vi "main.vi"(8 "Error in":errorcluster) -> (0 "error out":errorcluster)   [LabVIEW 2018, in "Sensor Interface.lvlib"]
doc: "The main VI of the module."
uses:
  Sensor Interface.lvlib
  vi/Module Queue Actions.ctl
  ctl/Module State--enum.ctl
  Common/Common.lvlib
  Common/ctl/Stop all modules states--enum.ctl
  Error Handler/Error Handler.lvlib
  Error Handler/ctl/Module State--enum.ctl
  Error Handler/ctl/Error source--enum.ctl
  Common/ctl/Error to pass.ctl
  Controller/Controller.lvlib
  Controller/ctl/Module State--enum.ctl
panel:
  in  "Funds Dispensed":bool
  in  "Deposit Received":bool
  # "Sensor Interface"
  # "[Covers: UI1]"
  # "[Covers: UI4]"
  # "[Covers: UI4A]"
  # "[Covers: UI4B]"
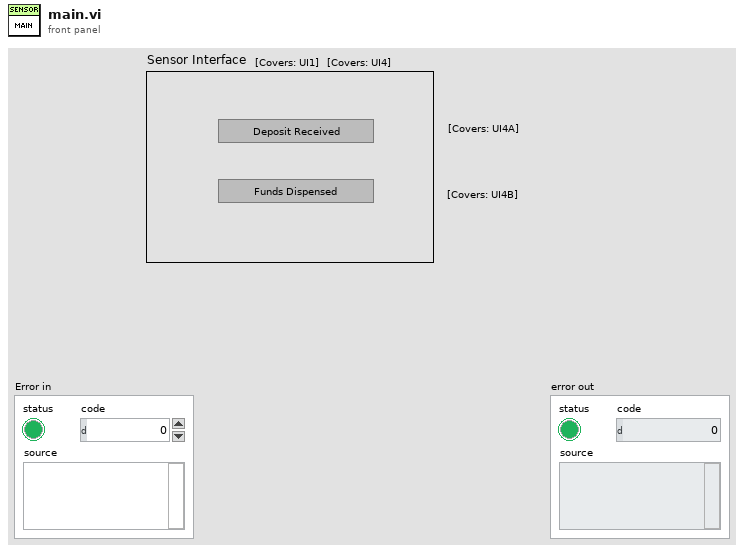
[diagram p1: front panel]
types:
  T1 = typedef "Sensor Interface.lvlib/Module Queue Actions.ctl" = enum16{"Create", "Get", "Destroy"}
  T2 = typedef "Common.lvlib/Stop all modules states--enum.ctl" = enum16{"Create", "Get", "Send 'Stop all' Message", "Destroy"}
  T3 = typedef "Sensor Interface.lvlib/Module State--enum.ctl" = enum16{"Init", "Error", "Idle", "Close", "Enable/disable controls"}
  T4 = typedef "Common.lvlib/Error source--enum.ctl" = enum16{"Display Console", "User Console", "Sensor Interface IO", "Process Step", "Other"}
  T5 = typedef "Common.lvlib/Error to pass.ctl" = cluster{"Error source":T4, "Error":errorcluster}
  T6 = typedef "Error Handler.lvlib/Module State--enum.ctl" = enum16{"Init", "Error", "Idle", "Close", "Handle External Error", "Log to file"}
  T7 = typedef "Controller.lvlib/Module State--enum.ctl" = enum16{"Init", "Error", "Close", "User Console: Card Reader Pressed", "Sensor Interface: Deposit Received pressed", "Sensor Interface: Funds Dispensed Pressed", "Idle", "Login State", "Balance Enquiry", "Deposit State", "Withdrawal State", "Fast Cash State", "Configuration Database", "Inactivity Timeout", "Terminate State", "Wait for account number", "Verify account number", "Wait for new transaction button"}
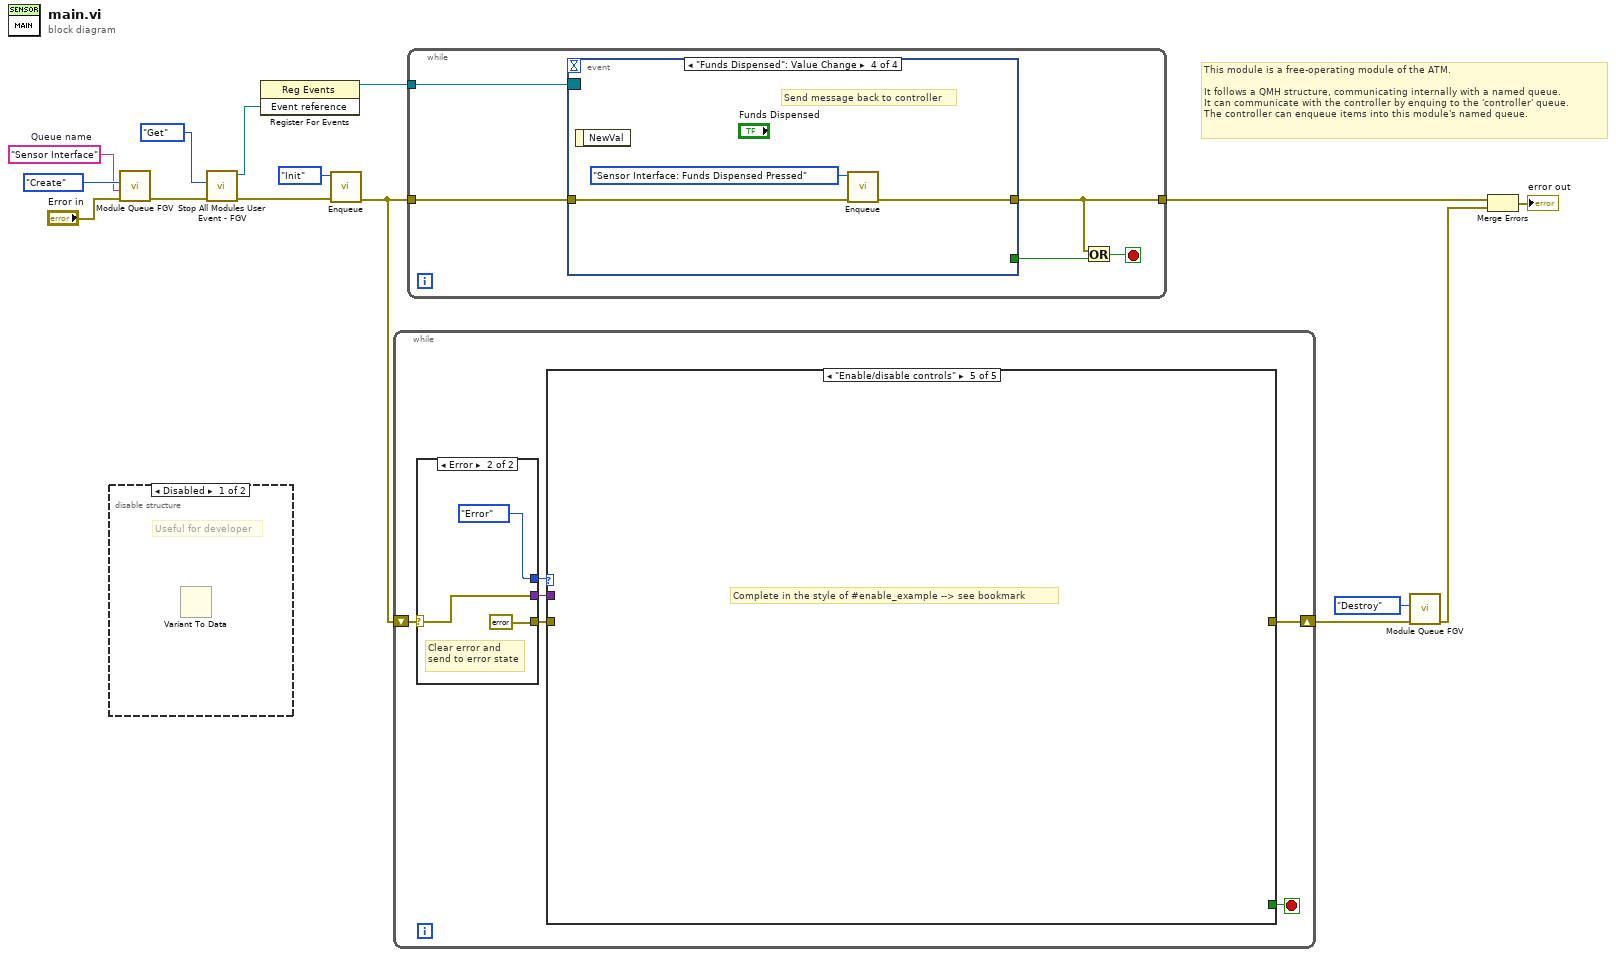
[diagram p0: block diagram]
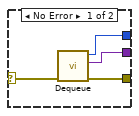
[diagram p3: hidden frame]
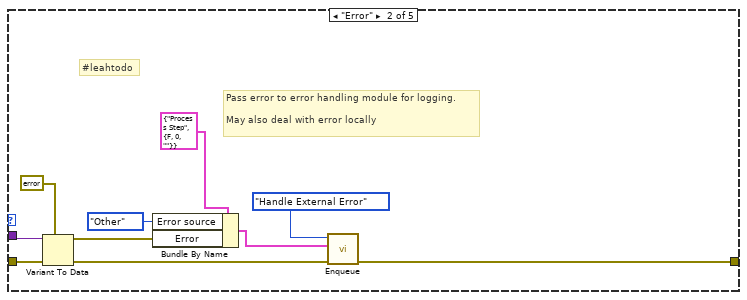
[diagram p5: hidden frame]
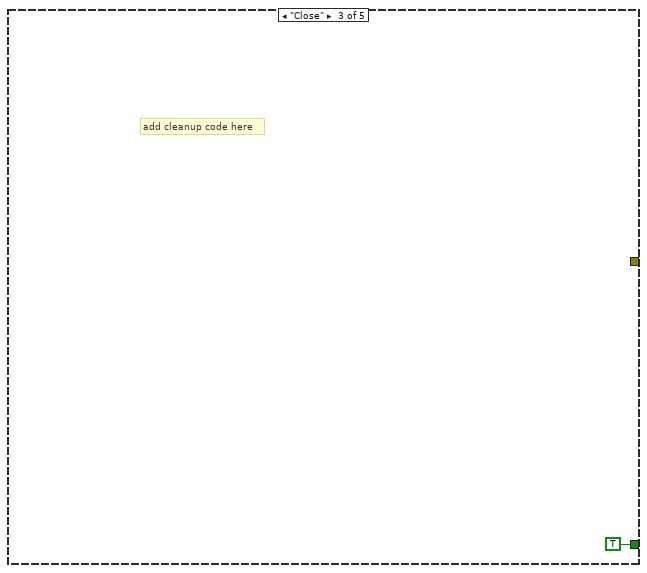
[diagram p6: hidden frame]
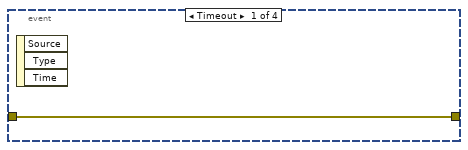
[diagram p8: hidden frame]
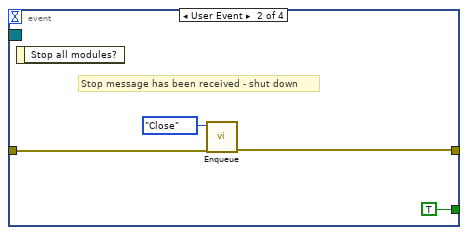
[diagram p9: hidden frame]
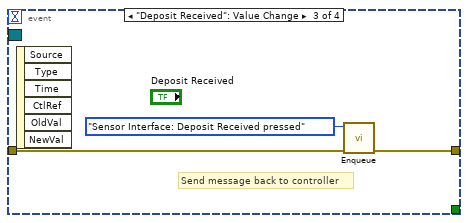
[diagram p10: hidden frame]
diagram:
  w14 = "Sensor Interface"  # Queue name
  # "This module is a free-operating module of the ATM.\n\nIt follows a QMH structure, communicating internally with a named queue.\nIt can communicate with the controller by enquing to the 'controller' queue.\nThe controller can enqueue items into this module's named queue."
  n1 = disable-structure shown="Disabled" {
    frame Disabled {
      # "Useful for developer"
      n2 = Variant To Data() -> ()  [unwired: 3 in, 2 out]
    }
    frame Enabled {
    }
  }
  n3 = call "Module Queue FGV.vi"("Error in"="Error in", "Queue name"=w14, "Module Queue Actions"=Module_Queue_Actions."Create") -> ("error out"=w9:errorcluster)  [unwired: 7 in, 1 out]
  n4 = call "Stop All Modules User Event - FGV.vi"("error in"=w9, "Action"=Stop_all_modules_states--enum."Get") -> ("error out"=w8:errorcluster, "Event reference"=w11:refnum<user-event>)  [unwired: 8 in]
  n5 = register-events(w11) -> (reference out=w10:refnum<event-registration>)  [unwired: 2 in, 1 out]
  n6 = call "Enqueue.vi"("error in (no error)"=w8, "State"=Module_State--enum."Init") -> ("error out"=w7:errorcluster)  [unwired: 9 in]
  n7 = while {
    shift-right: [w18] -> w5
    shift-left: w7 -> [w17]
    stop <- w16 stop-if-true
    n8 = case shown="Error" w17 {
      selector: w17 -> [w22 w27]
      tunnel: [w25 Module_State--enum."Error" ("State")] -> w21
      tunnel: [w24 w27] -> w20
      tunnel: [w23 errorcluster {"status"=FALSE, "code"=0, "source"=""} ("error out")] -> w19
      frame No Error {
        n9 = call "Dequeue.vi"("error in (no error)"=w22) -> ("error out"=w23:errorcluster, "Data"=w24:variant, "State"=w25:T3)  [unwired: 8 in]
      }
      frame Error {
        # "Clear error and\nsend to error state"
      }
    }
    n10 = case shown="\"Enable/disable controls\"" w21 {
      tunnel: w20 -> [_ w35 _ _ _]
      tunnel: w19 -> [_ w36 _ _ _]
      tunnel: [_ w37 _ _ _] -> w18
      tunnel: [_ _ TRUE _ _] -> w16
      frame "Init", Default {
        # "Disable both controls"
        # "[Covers: IS3]"
      }
      frame "Error" {
        # "#leahtodo"
        # "Pass error to error handling module for logging.\n\nMay also deal with error locally"
        n11 = Variant To Data(error in=w36, type=errorcluster {"status"=FALSE, "code"=0, "source"=""} ("error constant"), Variant=w35) -> (data=w31:errorcluster, error out=w33:errorcluster)
        n12 = Bundle By Name(cluster=T5 {"Error source"=enum."Process Step", "Error"={"status"=FALSE, "code"=0, "source"=""}} ("Error to pass"), "Error source"=Error_source--enum."Other", "Error"=w31) -> (w30:T5)
        n13 = call "Enqueue.vi"("error in (no error)"=w33, "Data"=w30, "State"=Module_State--enum."Handle External Error") -> ("error out"=w37:errorcluster)  [unwired: 8 in]
      }
      frame "Close" {
        # "add cleanup code here"
      }
      frame "Idle" {
      }
      frame "Enable/disable controls" {
        # "Complete in the style of #enable_example --> see bookmark"
      }
    }
  }
  n14 = while {
    tunnel: w7 -> [w44]
    tunnel: [w41] -> w3
    tunnel: w10 -> [w43]
    stop <- w42 stop-if-true
    n15 = event shown="[3] \"Funds Dispensed\": Value Change" {
      selector: w43 -> [_ _ _ _]
      dyn-events: _ -> [_ _ _ _]
      timeout: _ -> [_ _ _ _]
      tunnel: w44 -> [w45 w49 w51 w54]
      tunnel: [w45 w48 w50 w53] -> w41
      tunnel: [_ TRUE _ _] -> w40
      event Timeout {
        n16 = event-data() -> ()  [unwired: 1 in, 3 out]
      }
      event User Event {
        # "Stop message has been received - shut down"
        n17 = event-data() -> ()  [unwired: 1 in, 1 out]
        n18 = call "Enqueue.vi"("error in (no error)"=w49, "State"=Module_State--enum."Close") -> ("error out"=w48:errorcluster)  [unwired: 9 in]
      }
      event "Deposit Received": Value Change {
        # "Send message back to controller"
        n19 = event-data() -> ()  [unwired: 1 in, 6 out]
        n20 = call "Enqueue.vi"("error in (no error)"=w51, "State"=Module_State--enum."Sensor Interface: Deposit Received pressed") -> ("error out"=w50:errorcluster)  [unwired: 9 in]
      }
      event "Funds Dispensed": Value Change {
        # "Send message back to controller"
        n21 = event-data() -> ()  [unwired: 1 in, 1 out]
        n22 = call "Enqueue.vi"("error in (no error)"=w54, "State"=Module_State--enum."Sensor Interface: Funds Dispensed Pressed") -> ("error out"=w53:errorcluster)  [unwired: 9 in]
      }
    }
    n23 = Or(x=w41, y=w40) -> (x .or. y?=w42:bool)
  }
  n24 = call "Module Queue FGV.vi"("Error in"=w5, "Module Queue Actions"=Module_Queue_Actions."Destroy") -> ("error out"=w4:errorcluster)  [unwired: 8 in, 1 out]
  n25 = Merge Errors(w3, w4) -> (→"error out":errorcluster)
